vi "Create TOC Line.vi"(0 "PDF Report IN":refnum<class "PDF Report Class.lvclass">, 2 "Indentation (points)":T1=36.0, 5 "Font Ref":refnum<k24>, 7 "Font Size":T1=12.0, 9 "Width (points)":sgl, 11 "error in (no error)":errorcluster, 13 "TOC Line":T2={"Title"="", "Level"=0, "GoTo Page"=0, "GoTo Position"=0, "Destination"="", "Type & run direction"=enum."UTF-16"}) -> (4 "PDF Report OUT":refnum<class "PDF Report Class.lvclass">, 8 "Paragraph":refnum<k24>, 15 "error out":errorcluster)   [LabVIEW 2020, in "Exaprom PDF.lvlib"]
doc: "Version 1.1\nDeveloped by Jean-Marc Simard\nCopyright © 2012, Exaprom Inc.\nAll rights reserved.\nLicense: BSD\n\nWith iTextSharp 4.1.6 (http://itextsharp.sourceforge.net)\nunder Mozilla Public License Version 1.1\n(http://www.mozilla.org/MPL/MPL-1.1.html)"
uses:
  <userlib>/labview-PDF-writer-master/Exaprom PDF.lvlib
  <userlib>/labview-PDF-writer-master/LV Class/PDF Report Class/PDF Report Class.lvclass
  <userlib>/labview-PDF-writer-master/Controls/Chapter Controls/TOC Line.ctl
  <userlib>/labview-PDF-writer-master/Controls/Text Controls/Unicode/Type and run direction.ctl
  C:/Program Files (x86)/National Instruments/LabVIEW 2020/user.lib/labview-PDF-writer-master/DLL/itextsharp.dll
  DLL/itextsharp.dll
  <userlib>/labview-PDF-writer-master/Controls/Font Controls/Font size.ctl
panel:
  # "缩进"
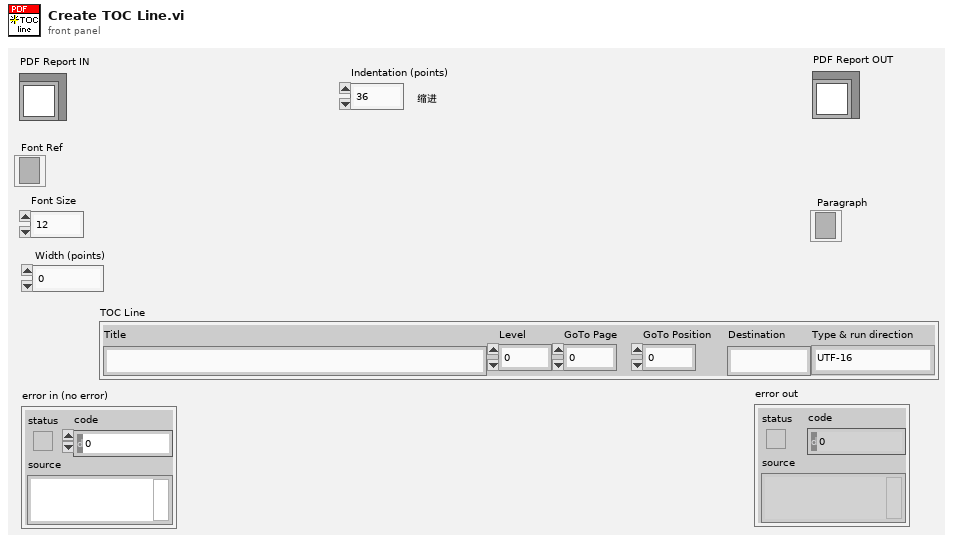
[diagram p1: front panel]
types:
  T1 = typedef "Exaprom PDF.lvlib/Font size.ctl" = sgl
  T2 = typedef "Exaprom PDF.lvlib/TOC Line.ctl" = cluster{"Title":string, "Level":u16, "GoTo Page":u16, "GoTo Position":u16, "Destination":string, "Type & run direction":T3}
  T3 = typedef "Exaprom PDF.lvlib/Type and run direction.ctl" = enum16{"Select", "ASCII", "UTF-16", "UTF-16 (default)", "UTF-16 (LTR)", "UTF-16 (RTL)"}
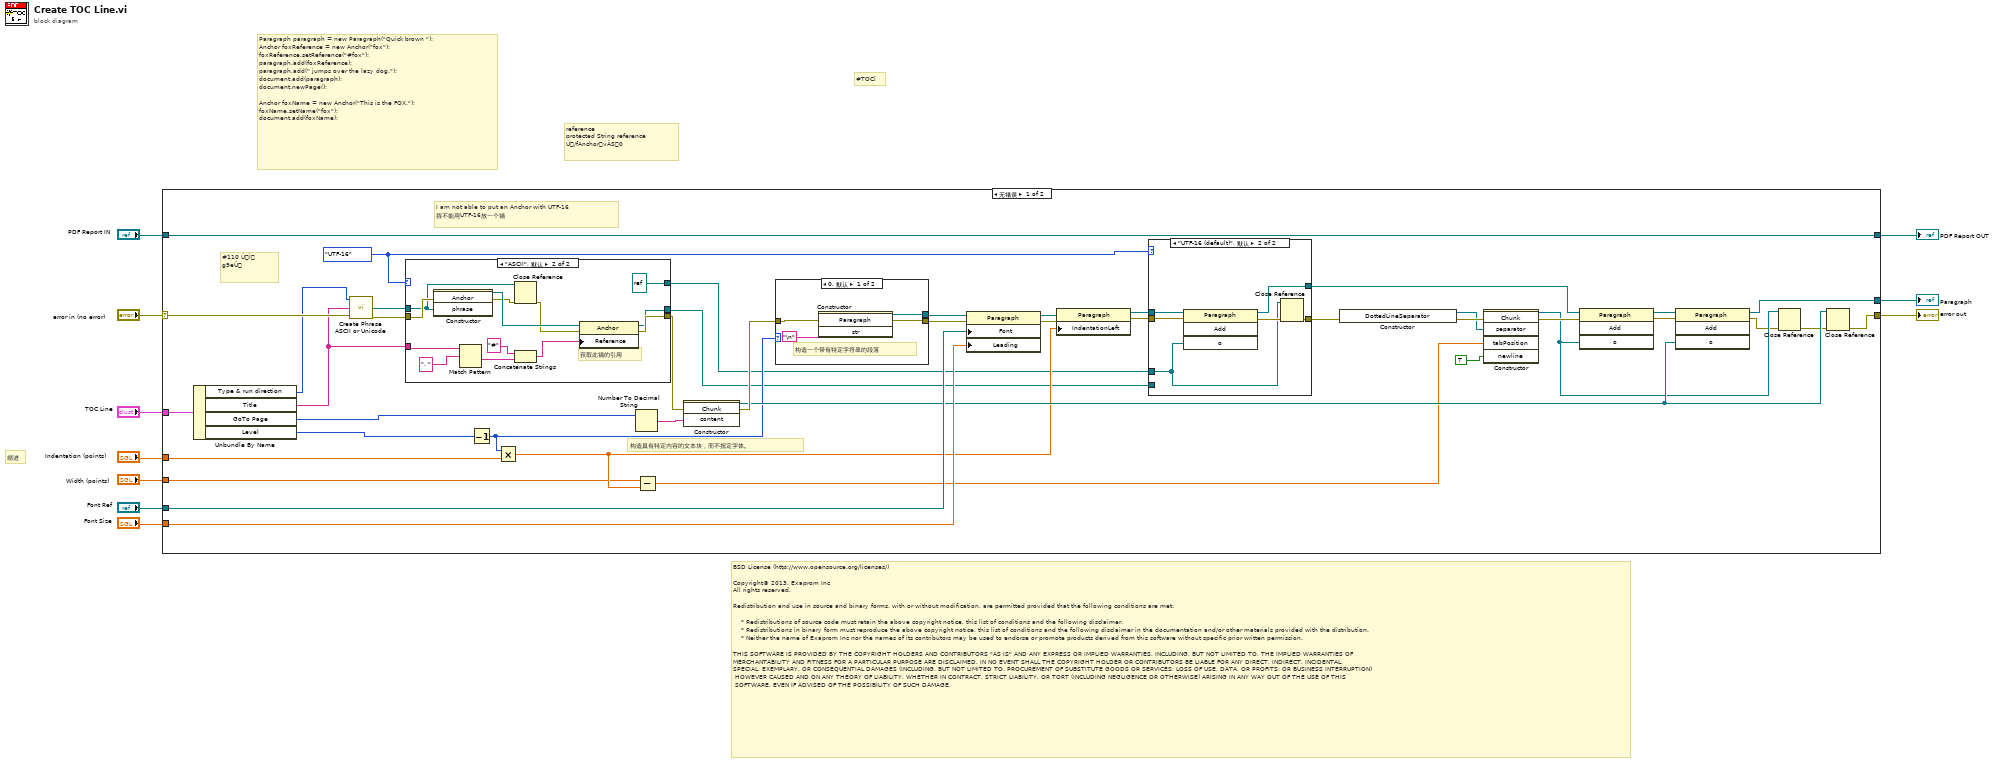
[diagram p0: block diagram]
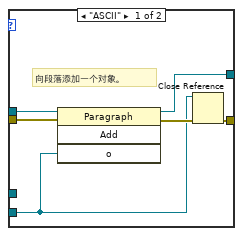
[diagram p2: hidden frame]
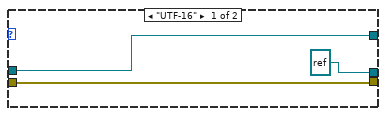
[diagram p3: hidden frame]
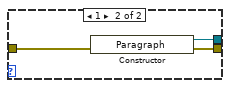
[diagram p4: hidden frame]
diagram:
  # "#TOCî"
  # "reference\nprotected String reference\nÙ/fAnchorvÂS0"
  # "缩进"
  # "Paragraph paragraph = new Paragraph(\"Quick brown \");\nAnchor foxReference = new Anchor(\"fox\");\nfoxReference.setReference(\"#fox\");\nparagraph.add(foxReference);\nparagraph.add(\" jumps over the lazy dog.\");\ndocument.add(paragraph);\ndocument.newPage();\n\nAnchor foxName = new Anchor(\"This is the FOX.\");\nfoxName.setName(\"fox\");\ndocument.add(foxName);"
  # "BSD License (http://www.opensource.org/licenses/)\n\nCopyright© 2013, Exaprom Inc\nAll rights reserved.\n\nRedistribution and use in source and binary forms, with or without modification, are permitted provided that the following conditions are met:\n\n    * Redistributions of source code must retain the above copyright notice, this list of conditions and the following disclaimer.\n    * Redistributions in binary form must reproduce the above copyright notice, this list of conditions and the following disclaimer in the documentation and/or other materials provided with the distribution.\n    * Neither the name of Exaprom Inc nor the names of its contributors may be used to endorse or promote products derived from this software without specific prior written permission.\n\nTHIS SOFTWARE IS PROVIDED BY THE COPYRIGHT HOLDERS AND CONTRIBUTORS \"AS IS\" AND ANY EXPRESS OR IMPLIED WARRANTIES, INCLUDING, BUT NOT LIMITED TO, THE IMPLIED WARRANTIES OF \nMERCHANTABILITY AND FITNESS FOR A PARTICULAR PURPOSE ARE DISCLAIMED. IN NO EVENT SHALL THE COPYRIGHT HOLDER OR CONTRIBUTORS BE LIABLE FOR ANY DIRECT, INDIRECT, INCIDENTAL,\nSPECIAL, EXEMPLARY, OR CONSEQUENTIAL DAMAGES (INCLUDING, BUT NOT LIMITED TO, PROCUREMENT OF SUBSTITUTE GOODS OR SERVICES; LOSS OF USE, DATA, OR PROFITS; OR BUSINESS INTERRUPTION)\n HOWEVER CAUSED AND ON ANY THEORY OF LIABILITY, WHETHER IN CONTRACT, STRICT LIABILITY, OR TORT (INCLUDING NEGLIGENCE OR OTHERWISE) ARISING IN ANY WAY OUT OF THE USE OF THIS\n SOFTWARE, EVEN IF ADVISED OF THE POSSIBILITY OF SUCH DAMAGE."
  n1 = case shown="无错误" "error in (no error)" {
    selector: "error in (no error)" -> [w23 w88]
    tunnel: "PDF Report IN" -> [w52 w89]
    tunnel: [w52 w89] -> w9
    tunnel: [w43 w88] -> w8
    tunnel: "TOC Line" -> [w45 _]
    tunnel: "Width (points)" -> [w24 _]
    tunnel: "Font Ref" -> [w42 _]
    tunnel: "Font Size" -> [w41 _]
    tunnel: [w40 _] -> w2
    tunnel: "Indentation (points)" -> [w34 _]
    frame No Error {
      w11 = Type_and_run_direction."UTF-16" ("Type & run direction")
      # "#110 ÙÌ\tg9eÛ"
      # "构造具有特定内容的文本块，而不指定字体。"
      # "I am not able to put an Anchor with UTF-16\n我不能用UTF-16放一个锚"
      n2 = Unbundle By Name(w45) -> ("Type & run direction"=w12:T3, "Title"=w17:string, "GoTo Page"=w50:u16, "Level"=w35:u16)
      n3 = call <userlib>:"Create Phrase ASCII or Unicode.vi"("Character type"=w12, "Text"=w17, "error in (no error)"=w23) -> ("Phrase refnum"=w18:refnum<k24>, "error out"=w20:errorcluster)  [unwired: 10 in, 1 out]
      n4 = case shown="\"ASCII\", 默认" w11 {
        tunnel: w20 -> [w66 w79]
        tunnel: [w66 w78] -> w19
        tunnel: w18 -> [w65 w74]
        tunnel: w17 -> [_ w71]
        tunnel: [refnum<k24> refnum ("new reference") w70] -> w15
        tunnel: [w65 refnum<k24> refnum ("Phrase refnum")] -> w13
        frame "UTF-16" {
        }
        frame "ASCII", Default {
          # "获取此锚的引用"
          n5 = constructor class="Anchor"(error in=w79, "phrase"=w74) -> (reference out=w80:refnum<k24>, error out=w76:errorcluster)  [unwired: 2 in, 2 out]
          n6 = Match Pattern(string=w71, regular expression=". ") -> (after substring=w72:string)  [unwired: 1 in, 3 out]
          n7 = Close Reference(reference=w74, error in (no error)=w76) -> (error out=w75:errorcluster)
          n8 = Concatenate Strings("#" ("string"), w72) -> (w68:string)
          n9 = property class="Anchor"(reference=w80, error in=w75, "Reference"=w68) -> (reference out=w70:refnum<k24>, error out=w78:errorcluster)
        }
      }
      n10 = Decrement(x=w35) -> (x-1=w22:u16)
      n11 = Multiply(x=w22, y=w34) -> (x*y=w28:T1)
      n12 = Number To Decimal String(number=w50) -> (decimal integer string=w49:string)  [unwired: 1 in]
      n13 = Subtract(x=w24, y=w28) -> (x-y=w27:T1)
      n14 = constructor class="Chunk"(error in=w19, "content"=w49) -> (reference out=w33:refnum<k24>, error out=w44:errorcluster)  [unwired: 2 in, 2 out]
      n15 = case shown="0, 默认" w22 {
        tunnel: [w82 w87] -> w51
        tunnel: w44 -> [w84 w86]
        tunnel: [w83 w85] -> w26
        frame 0, Default {
          # "构造一个带有特定字符串的段落"
          n16 = constructor class="Paragraph"(error in=w84, "str"="\n") -> (reference out=w82:refnum<k24>, error out=w83:errorcluster)  [unwired: 2 in, 2 out]
        }
        frame 1 {
          n17 = constructor class="Paragraph"(error in=w86) -> (reference out=w87:refnum<k24>, error out=w85:errorcluster)  [unwired: 2 in, 1 out]
        }
      }
      n18 = property class="Paragraph"(reference=w51, error in=w26, "Font"=w42, "Leading"=w41) -> (reference out=w39:refnum<k24>, error out=w38:errorcluster)
      n19 = property class="Paragraph"(reference=w39, error in=w38, "IndentationLeft"=w28) -> (reference out=w36:refnum<k24>, error out=w37:errorcluster)
      n20 = case shown="\"UTF-16 (default)\", 默认" w11 {
        tunnel: [w58 w64] -> w48
        tunnel: w37 -> [w57 w63]
        tunnel: w36 -> [w56 w62]
        tunnel: [w54 w60] -> w16
        tunnel: w15 -> [w53 _]
        tunnel: w13 -> [_ w59]
        frame "ASCII" {
          # "向段落添加一个对象。"
          n21 = invoke class="Paragraph" method="Add"(reference=w56, error in=w57, "o"=w53) -> (reference out=w58:refnum<k24>, error out=w55:errorcluster)  [unwired: 1 in, 2 out]
          n22 = Close Reference(reference=w53, error in (no error)=w55) -> (error out=w54:errorcluster)
        }
        frame "UTF-16 (default)", Default {
          n23 = invoke class="Paragraph" method="Add"(reference=w62, error in=w63, "o"=w59) -> (reference out=w64:refnum<k24>, error out=w61:errorcluster)  [unwired: 1 in, 2 out]
          n24 = Close Reference(reference=w59, error in (no error)=w61) -> (error out=w60:errorcluster)
        }
      }
      n25 = constructor class="DottedLineSeparator"(error in=w16) -> (reference out=w31:refnum<k24>, error out=w32:errorcluster)  [unwired: 2 in, 1 out]
      n26 = constructor class="Chunk"(error in=w32, "separator"=w31, "tabPosition"=w27, "newline"=TRUE) -> (reference out=w21:refnum<k24>, error out=w29:errorcluster)  [unwired: 2 in, 4 out]
      n27 = invoke class="Paragraph" method="Add"(reference=w48, error in=w29, "o"=w21) -> (reference out=w47:refnum<k24>, error out=w46:errorcluster)  [unwired: 1 in, 2 out]
      n28 = invoke class="Paragraph" method="Add"(reference=w47, error in=w46, "o"=w33) -> (reference out=w40:refnum<k24>, error out=w14:errorcluster)  [unwired: 1 in, 2 out]
      n29 = Close Reference(reference=w21, error in (no error)=w14) -> (error out=w25:errorcluster)
      n30 = Close Reference(reference=w33, error in (no error)=w25) -> (error out=w43:errorcluster)
    }
    frame Error {
    }
  }
  "PDF Report OUT" <- w9
  "error out" <- w8
  "Paragraph" <- w2
